vi "update_attributes.vi"(8 "error in (no error)":errorcluster, 10 "Nested Enqueuers Map":T1(c390), 11 "UDP_transmitter in":refnum<class "UDP_transmitter.lvclass">) -> (0 "error out":errorcluster, 3 "UDP_transmitter out":refnum<class "UDP_transmitter.lvclass">)   [LabVIEW 2025, in "UDP_transmitter.lvlib" / "UDP_transmitter.lvclass"]
uses:
  UDP_transmitter.lvclass
  <vilib>/ActorFramework/Message Enqueuer/Message Enqueuer.lvclass
  UDP_transmitter.lvclass/UDP_transmitter.ctl
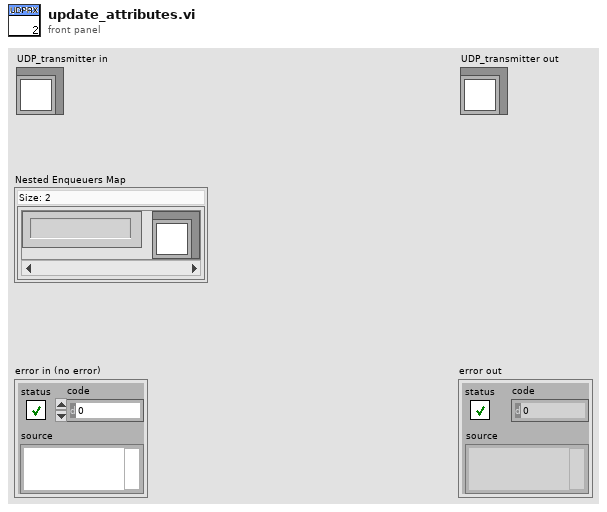
[diagram p1: front panel]
types:
  T1 = map{string, refnum<class "Message Enqueuer.lvclass">}
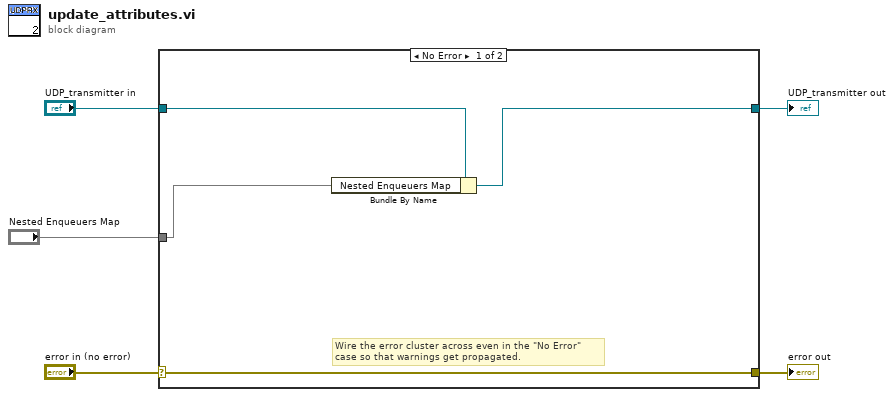
[diagram p0: block diagram]
diagram:
  n1 = case shown="No Error" "error in (no error)" {
    selector: "error in (no error)" -> [w9 w11]
    tunnel: [w9 w11] -> w1
    tunnel: [w6 w10] -> w3
    tunnel: "UDP_transmitter in" -> [w8 w10]
    tunnel: "Nested Enqueuers Map" -> [w7 _]
    frame No Error {
      # "Wire the error cluster across even in the \"No Error\"\ncase so that warnings get propagated."
      n2 = Bundle By Name(cluster=w8, "Nested Enqueuers Map"=w7) -> (w6:refnum<class "UDP_transmitter.lvclass">)
    }
    frame Error {
    }
  }
  "error out" <- w1
  "UDP_transmitter out" <- w3
